vi "ACT_Loop.vi"() -> ()   [LabVIEW 2023, in "Feeder_ACT.lvlib"]
uses:
  Feeder_ACT.lvlib
  Cluster_CMD_ACT_Data.ctl
  ENUM_CMD Mode.ctl
  ENUM_ACT_State.ctl
  <vilib>/Rock Robotics/WPI/PWM/Servo/WPI_ServoDeviceRef.ctl
  <vilib>/Rock Robotics/SystemInterfaces/DIO/FPGA_DIOPWMChannel.ctl
  <vilib>/Rock Robotics/WPI/PWM/WPI_PWMDeadband.ctl
  <vilib>/Rock Robotics/WPI/MotorControl/WPI_MotorControlDeviceRef.ctl
  <vilib>/Rock Robotics/WPI/MotorControl/WPI_MotorControlType.ctl
  <vilib>/Rock Robotics/SystemInterfaces/DIO/FPGA_DIOChannel.ctl
  <vilib>/Rock Robotics/WPI/DigitalInput/WPI_DigitalInputDevRef.ctl
  Shared Code/TypeDefs/ENUM RB_Feeder State.ctl
  ENUM_ACT_Action.ctl
  <vilib>/Rock Robotics/WPI/MotorControl/WPI_MotorControlOpen VictorSP.vi
  RoboRIO Utilities/Global_STOP.vi
  Global_CMD_ACT_Data In.vi
  Tube Wheel/Global_ACT_Data Out.vi
  Global_ACT_Data Out.vi
  Tube Wheel/Tube Wheel_ACT.lvlib
panel:
  out "State":T1
  out "Tube Wheel Ready":bool
  out "Puller Speed (0-1)":dbl
  out "Back":bool
  out "Input DBL Data":T2
  out "Pusher Position (0-100)":dbl
  out "Cycle Time (S)":dbl format="%.3g"
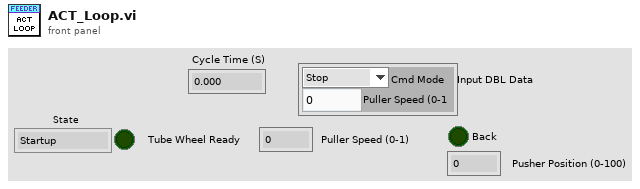
[diagram p1: front panel]
types:
  T1 = typedef "Feeder_ACT.lvlib/ENUM_ACT_State.ctl" = enum16{"Startup", "Back Waiting", "Push Feeding", "Retracting", "Shutdown"}
  T2 = typedef "Feeder_ACT.lvlib/Cluster_CMD_ACT_Data.ctl" = cluster{"Cmd Mode":T3, "Puller Speed (0-1":dbl}
  T3 = typedef "Feeder_ACT.lvlib/ENUM_CMD Mode.ctl" = enum16{"Stop", "Feed Pos 1", "Feed Pos 2", "Fead Full", "Back"}
  T4 = typedef "ENUM RB_Feeder State.ctl" = enum32{"Back", "Reversing", "Shooting"}
  T5 = typedef "WPI_DigitalInputDevRef.ctl" = cluster{"DevStatus":errorcluster, "DIO Channel":T6}
  T6 = typedef "FPGA_DIOChannel.ctl" = enum8{"DIO 0", "DIO 1", "DIO 2", "DIO 3", "DIO 4", "DIO 5", "DIO 6", "DIO 7", "DIO 8", "DIO 9", "DIO MXP 0", "DIO MXP 1", "DIO MXP 2", "DIO MXP 3", "DIO MXP 4", "DIO MXP 5", "DIO MXP 6", "DIO MXP 7", "DIO MXP 8", "DIO MXP 9", "DIO MXP 10", "DIO MXP 11", "DIO MXP 12", "DIO MXP 13", "DIO MXP 14", "DIO MXP 15", "SPI Port CS1", "SPI Port CS2", "SPI Port CS3", "SPI Port MISO", "SPI Port MOSI", "Invalid"}
  T7 = typedef "WPI_MotorControlDeviceRef.ctl" = cluster{"DeviceStatus":errorcluster, "Type":T8, "PWM":cluster{"PWM Channel":T9, "DeadBand":T10}, "CAN":cluster{"Device Number":u8, "SetOutput VI Ref":variant, "GetOutput VI Ref":variant, "Enable VI Ref":variant, "Disable VI Ref":variant, "Data":variant}, "Invert":bool, "DIO PWM":cluster{"PWM \"Enable\" Channel":T9, "DIOChannel":T6, "PWM Rate":dbl}}
  T8 = typedef "WPI_MotorControlType.ctl" = enum16{"PWM", "CAN", "DIO PWM"}
  T9 = typedef "FPGA_DIOPWMChannel.ctl" = enum8{"PWM 0", "PWM 1", "PWM 2", "PWM 3", "PWM 4", "PWM 5", "PWM 6", "PWM 7", "PWM 8", "PWM 9", "PWM MXP 0", "PWM MXP 1", "PWM MXP 2", "PWM MXP 3", "PWM MXP 4", "PWM MXP 5", "PWM MXP 6", "PWM MXP 7", "PWM MXP 8", "PWM MXP 9", "Invalid"}
  T10 = typedef "WPI_PWMDeadband.ctl" = cluster{"Name":string, "maxPositivePwm":i32, "minPositivePwm":i32, "centerPwm":i32, "maxNegativePwm":i32, "minNegativePwm":i32, "angularRange":u16}
  T11 = typedef "WPI_ServoDeviceRef.ctl" = cluster{"DeviceStatus":errorcluster, "PWM Channel":T9, "DeadBand":T10}
  T12 = typedef "Feeder_ACT.lvlib/ENUM_ACT_Action.ctl" = enum16{"No Action", "Reset Time", "Reset All", "Retract Back", "Set Push 1", "Set Push 2", "Set Push 3"}
  T13 = cluster{"PusherServo Ref":T11, "LeftMotor Puller Ref":T7, "RightMotor Puller Ref":T7, "PusherBack Ref":T5, "State":T1, "Previous State":T1, "Current Time":timestamp, "Previous Time":timestamp, "Start Time":timestamp, "Target Time (ms)":u32, "Cycle Time(S)":dbl, "ACT Input":T2, "Pusher Positon(0-100)":dbl, "Puller Speed (0-1)":dbl, "PusherIsBack":bool, "Feeder Display":T4, "Tube Wheel Ready":bool}
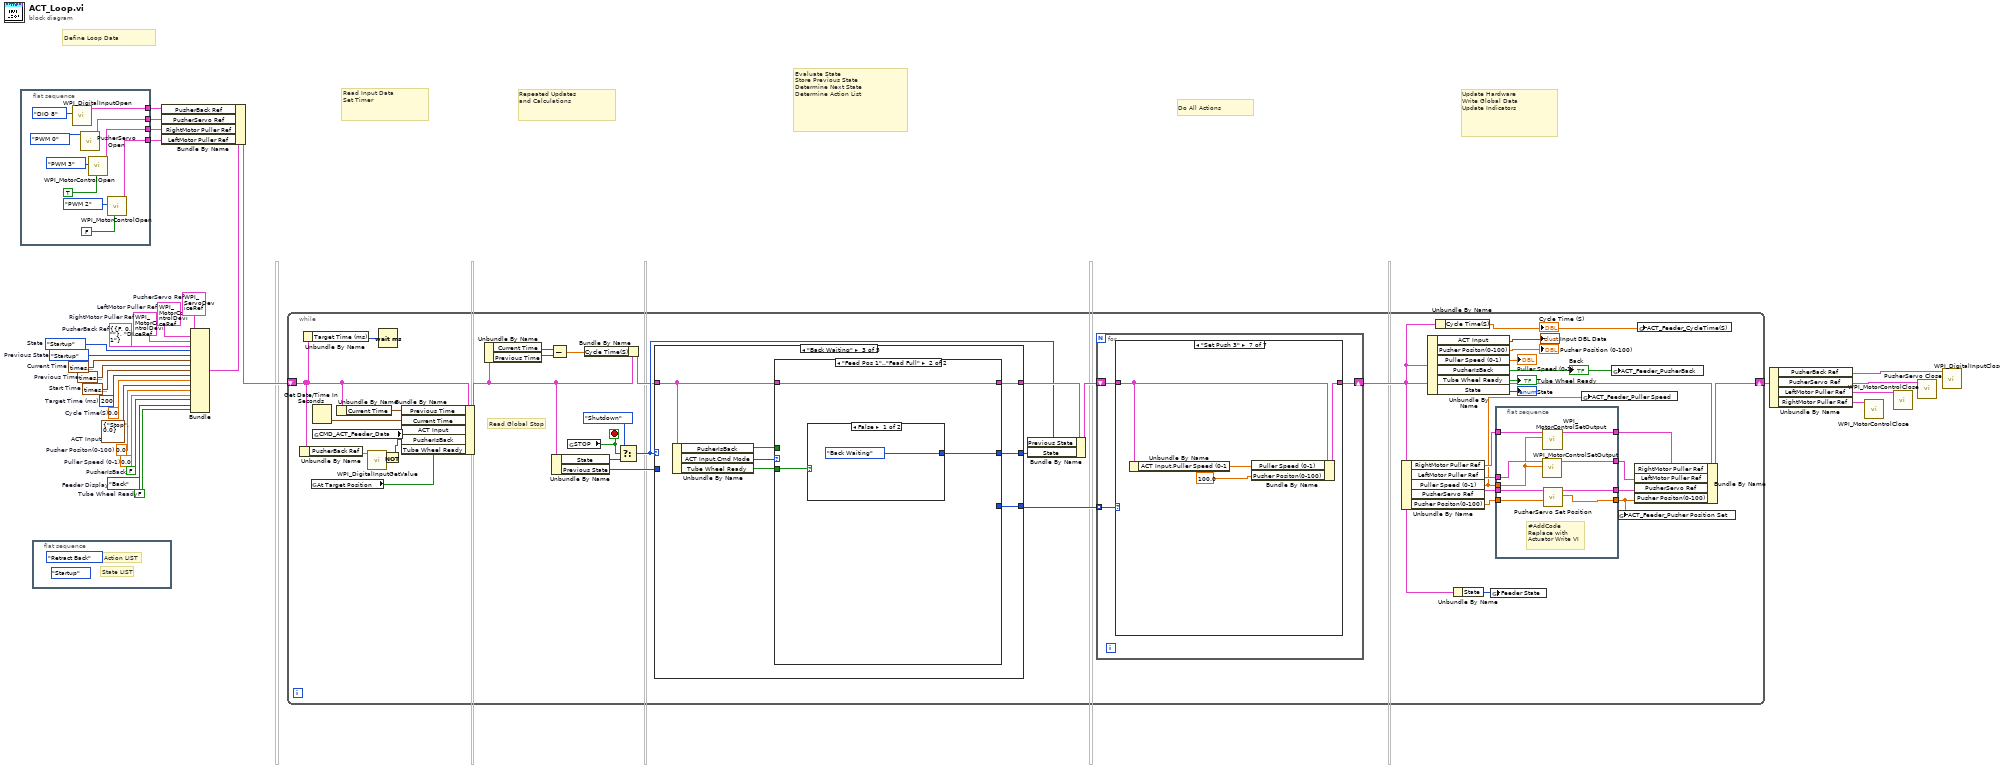
[diagram p0: block diagram]
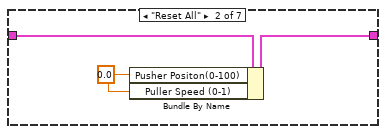
[diagram p3: hidden frame]
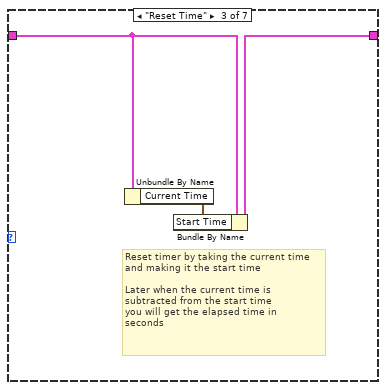
[diagram p4: hidden frame]
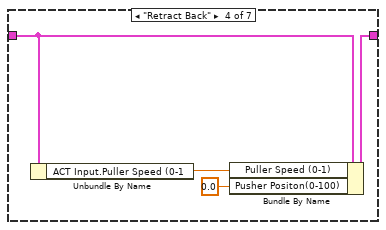
[diagram p5: hidden frame]
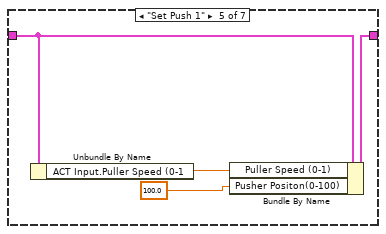
[diagram p6: hidden frame]
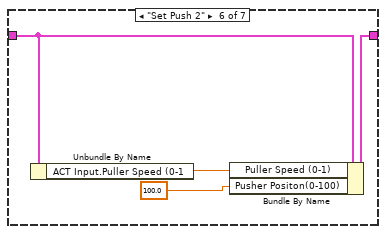
[diagram p7: hidden frame]
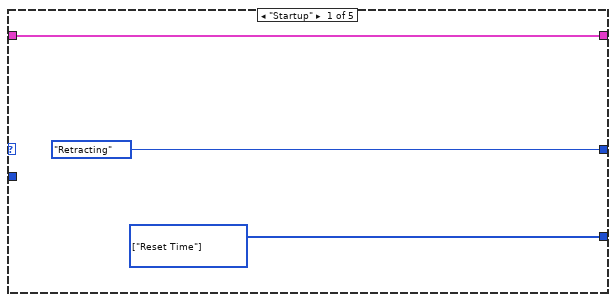
[diagram p8: hidden frame]
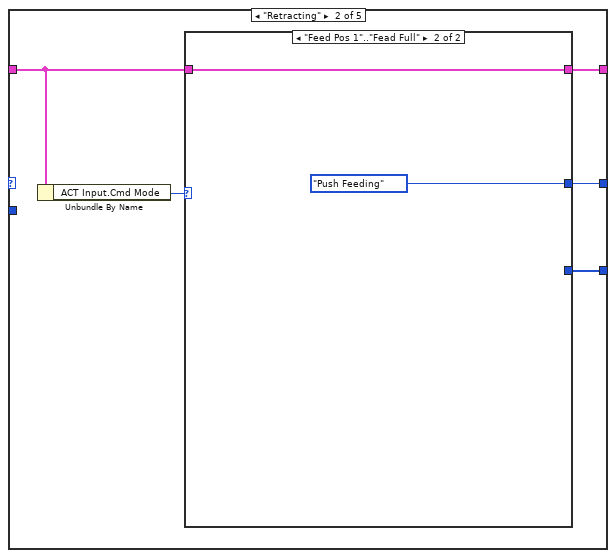
[diagram p9: hidden frame]
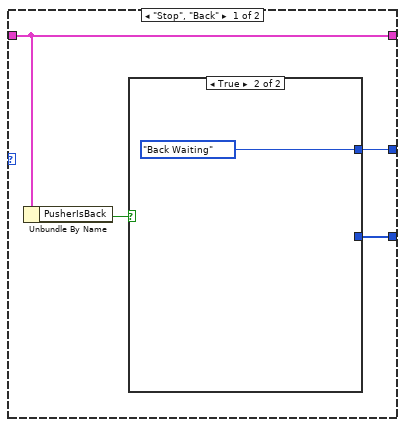
[diagram p10: hidden frame]
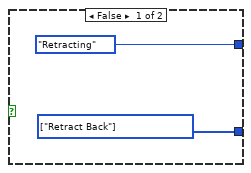
[diagram p11: hidden frame]
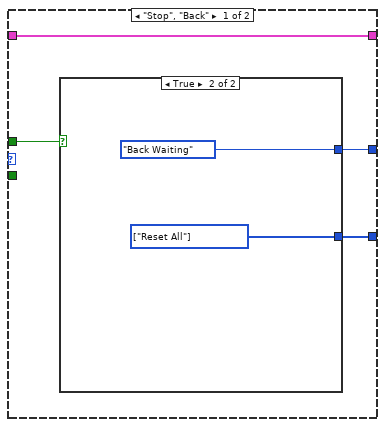
[diagram p12: hidden frame]
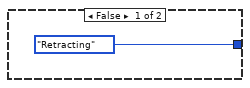
[diagram p13: hidden frame]
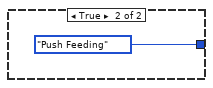
[diagram p14: hidden frame]
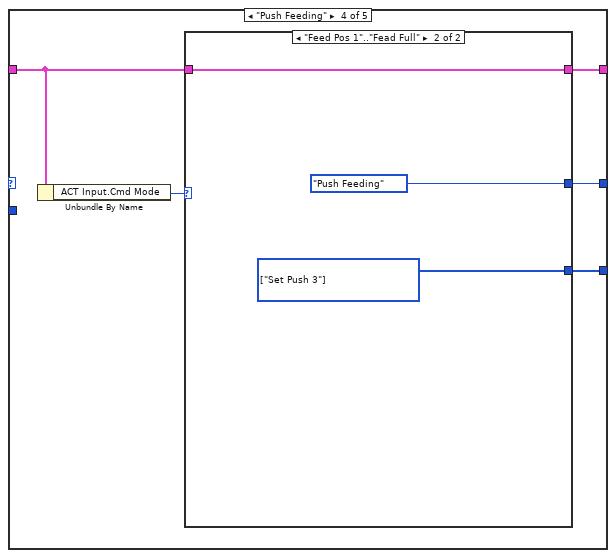
[diagram p15: hidden frame]
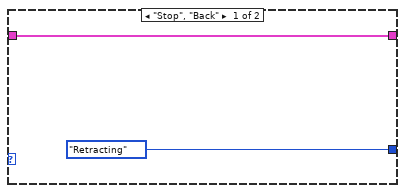
[diagram p16: hidden frame]
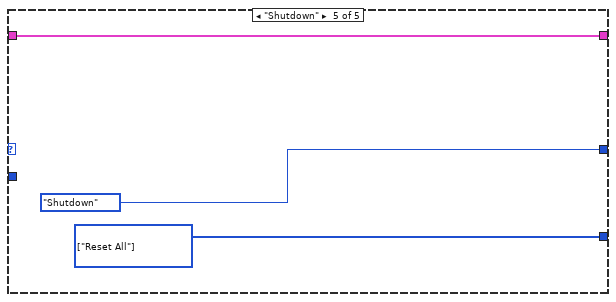
[diagram p17: hidden frame]
diagram:
  w1 = FALSE  # Tube Wheel Ready
  w2 = ENUM_RB_Feeder_State."Back"  # Feeder Display
  w4 = FALSE  # PusherIsBack
  w6 = T5 {"DevStatus"={"status"=FALSE, "code"=0, "source"=""}, "DIO Channel"=enum."DIO 1"}  # PusherBack Ref
  w7 = 0.0  # Puller Speed (0-1)
  w13 = T7 {"DeviceStatus"={"status"=FALSE, "code"=0, "source"=""}, "Type"=enum."PWM", "PWM"={"PWM Channel"=enum."Invalid", "DeadBand"={"Name"="", "maxPositivePwm"=0, "minPositivePwm"=0, "centerPwm"=0, "maxNegativePwm"=0, "minNegativePwm"=0, "angularRange"=0}}, "CAN"={"Device Number"=0, "SetOutput VI Ref"=variant(refnum<vi> refnum), "GetOutput VI Ref"=variant(refnum<vi> refnum), "Enable VI Ref"=variant(refnum<vi> refnum), "Disable VI Ref"=variant(refnum<vi> refnum), "Data"=variant}, "Invert"=FALSE, "DIO PWM"={"PWM \"Enable\" Channel"=enum."Invalid", "DIOChannel"=enum."Invalid", "PWM Rate"=0.0}}  # RightMotor Puller Ref
  w12 = T7 {"DeviceStatus"={"status"=FALSE, "code"=0, "source"=""}, "Type"=enum."PWM", "PWM"={"PWM Channel"=enum."Invalid", "DeadBand"={"Name"="", "maxPositivePwm"=0, "minPositivePwm"=0, "centerPwm"=0, "maxNegativePwm"=0, "minNegativePwm"=0, "angularRange"=0}}, "CAN"={"Device Number"=0, "SetOutput VI Ref"=variant(refnum<vi> refnum), "GetOutput VI Ref"=variant(refnum<vi> refnum), "Enable VI Ref"=variant(refnum<vi> refnum), "Disable VI Ref"=variant(refnum<vi> refnum), "Data"=variant}, "Invert"=FALSE, "DIO PWM"={"PWM \"Enable\" Channel"=enum."Invalid", "DIOChannel"=enum."Invalid", "PWM Rate"=0.0}}  # LeftMotor Puller Ref
  w15 = T11 {"DeviceStatus"={"status"=FALSE, "code"=0, "source"=""}, "PWM Channel"=enum."Invalid", "DeadBand"={"Name"="", "maxPositivePwm"=0, "minPositivePwm"=0, "centerPwm"=0, "maxNegativePwm"=0, "minNegativePwm"=0, "angularRange"=0}}  # PusherServo Ref
  w20 = 0.0  # Cycle Time(S)
  w21 = ENUM_ACT_State."Startup"  # Previous State
  w22 = timestamp(0 s since 1904-01-01)  # Previous Time
  w23 = u32 200  # Target Time (ms)
  w24 = 0.0  # Pusher Positon(0-100)
  w25 = T2 {"Cmd Mode"=enum."Stop", "Puller Speed (0-1"=0.0}  # ACT Input
  w26 = timestamp(0 s since 1904-01-01)  # Start Time
  w27 = timestamp(0 s since 1904-01-01)  # Current Time
  w28 = ENUM_ACT_State."Startup"  # State
  # "Define Loop Data"
  # "Repeated Updates\nand Calculations"
  # "Read Input Data\nSet Timer"
  # "Evaluate State\nStore Previous State\nDetermine Next State\nDetermine Action List"
  # "Do All Actions"
  # "Update Hardware\nWrite Global Data\nUpdate Indicators"
  n1 = flat-sequence {
    tunnel: [w37] -> w16
    tunnel: [w34] -> w11
    tunnel: [w31] -> w10
    tunnel: [w30] -> w5
    frame #0 {
      n2 = call <vilib>:"WPI_DigitalInputOpen.vi"("DIO Channel"=FPGA_DIOChannel."DIO 8") -> ("DigitalInputDevRef"=w30:T5)  [unwired: 9 in, 1 out]
      n3 = call "PusherServo Open.vi"("PWM Channel"=FPGA_DIOPWMChannel."PWM 0") -> ("ServoDeviceRef Out"=w37:T11)  [unwired: 9 in, 1 out]
      n4 = call-poly <vilib>:"WPI_MotorControlOpen.vi"("Invert"=TRUE, "PWM Channel"=FPGA_DIOPWMChannel."PWM 3") -> ("MotorControlDeviceRef"=w34:T7)  [unwired: 8 in, 1 out]
      n5 = call-poly <vilib>:"WPI_MotorControlOpen.vi"("Invert"=FALSE, "PWM Channel"=FPGA_DIOPWMChannel."PWM 2") -> ("MotorControlDeviceRef"=w31:T7)  [unwired: 8 in, 1 out]
    }
  }
  n6 = flat-sequence {
    frame #0 {
      (unwired) ENUM_ACT_State."Startup" ("State")
      (unwired) ENUM_ACT_Action."Retract Back" ("Action")
      # "State LIST"
      # "Action LIST"
    }
  }
  n7 = Bundle("PusherServo Ref"=w15, "LeftMotor Puller Ref"=w12, "RightMotor Puller Ref"=w13, "PusherBack Ref"=w6, "State"=w28, "Previous State"=w21, "Current Time"=w27, "Previous Time"=w22, "Start Time"=w26, "Target Time (ms)"=w23, "Cycle Time(S)"=w20, "ACT Input"=w25, "Pusher Positon(0-100)"=w24, "Puller Speed (0-1)"=w7, "PusherIsBack"=w4, "Feeder Display"=w2, "Tube Wheel Ready"=w1) -> (w18:T13)  [unwired: 1 in]
  n8 = Bundle By Name(cluster=w18, "PusherBack Ref"=w5, "PusherServo Ref"=w16, "RightMotor Puller Ref"=w11, "LeftMotor Puller Ref"=w10) -> (w17:T13)
  n9 = while {
    shift-right: [w58] -> w19
    shift-left: w17 -> [w50]
    stop <- w76 stop-if-true
    # "Read Global Stop"
    n10 = Unbundle By Name(w50) -> ("PusherBack Ref"=w49:T5)
    n11 = Unbundle By Name(w50) -> ("Target Time (ms)"=w73:u32)
    n12 = global read "Global_ACT_Data Out.vi" "At Target Position"() -> (w41:bool)
    n13 = Get Date/Time In Seconds() -> (seconds since 1Jan1904=w80:timestamp)
    n14 = global read "Global_CMD_ACT_Data In.vi" "CMD_ACT_Feeder_Data"() -> (w61:T2)
    n15 = Unbundle By Name(w50) -> ("Current Time"=w72:timestamp)
    n16 = call <vilib>:"WPI_DigitalInputGetValue.vi"("DigitalInputDevRef"=w49) -> ("Value"=w48:bool)  [unwired: 8 in, 2 out]
    n17 = Wait (ms)(milliseconds to wait=w73) -> ()  [unwired: 1 out]
    n18 = Not(x=w48) -> (.not. x?=w47:bool)
    n19 = Bundle By Name(cluster=w50, "Previous Time"=w72, "Current Time"=w80, "ACT Input"=w61, "PusherIsBack"=w47, "Tube Wheel Ready"=w41) -> (w66:T13)
    n20 = Unbundle By Name(w66) -> ("Current Time"=w67:timestamp, "Previous Time"=w68:timestamp)
    n21 = Subtract(x=w67, y=w68) -> (x-y=w64:dbl)
    n22 = Unbundle By Name(w66) -> ("State"=w74:T1, "Previous State"=w71:T1)
    n23 = global read "Global_STOP.vi" "STOP"() -> (w76:bool)
    n24 = Bundle By Name(cluster=w66, "Cycle Time(S)"=w64) -> (w65:T13)
    n25 = Select(t=ENUM_ACT_State."Shutdown" ("State"), s=w76, f=w74) -> (s? t:f=w69:T1)
    n26 = case shown="\"Back Waiting\"" w69 {
      tunnel: w65 -> [w118 w121 w137 w154 w164]
      tunnel: [w118 w120 w136 w153 w164] -> w78
      tunnel: [ENUM_ACT_State."Retracting" ("State") w123 w139 w156 ENUM_ACT_State."Shutdown" ("State")] -> w77
      tunnel: [w117 w119 w135 w152 w162] -> w63
      tunnel: w71 -> [_ _ _ _ _]
      frame "Startup" {
        w117 = T12[] [enum."Reset Time"] items=["No Action", "Reset Time", "Reset All", "Retract Back", "Set Push 1", "Set Push 2", "Set Push 3"] ("Actions")
      }
      frame "Retracting" {
        n27 = Unbundle By Name(w121) -> ("ACT Input.Cmd Mode"=w122:T3)
        n28 = case shown="\"Feed Pos 1\"..\"Fead Full\"" w122 {
          tunnel: [w127 ENUM_ACT_State."Push Feeding" ("State")] -> w123
          tunnel: w121 -> [w126 w131]
          tunnel: [w126 w131] -> w120
          tunnel: [w124 _] -> w119
          frame "Stop", "Back" {
            n29 = Unbundle By Name(w126) -> ("PusherIsBack"=w125:bool)
            n30 = case shown="True" w125 {
              tunnel: [ENUM_ACT_State."Retracting" ("State") ENUM_ACT_State."Back Waiting" ("State")] -> w127
              tunnel: [w128 _] -> w124
              frame False {
                w128 = T12[] [enum."Retract Back"] items=["No Action", "Reset Time", "Reset All", "Retract Back", "Set Push 1", "Set Push 2", "Set Push 3"] ("Actions")
              }
              frame True {
              }
            }
          }
          frame "Feed Pos 1".."Fead Full" {
          }
        }
      }
      frame "Back Waiting" {
        n31 = Unbundle By Name(w137) -> ("PusherIsBack"=w134:bool, "ACT Input.Cmd Mode"=w138:T3, "Tube Wheel Ready"=w133:bool)
        n32 = case shown="\"Feed Pos 1\"..\"Fead Full\"" w138 {
          tunnel: [w143 w149] -> w139
          tunnel: w137 -> [w142 w148]
          tunnel: [w142 w148] -> w136
          tunnel: [w141 _] -> w135
          tunnel: w134 -> [w140 _]
          tunnel: w133 -> [_ w147]
          frame "Stop", "Back" {
            n33 = case shown="True" w140 {
              tunnel: [ENUM_ACT_State."Retracting" ("State") ENUM_ACT_State."Back Waiting" ("State")] -> w143
              tunnel: [_ w145] -> w141
              frame False {
              }
              frame True {
                w145 = T12[] [enum."Reset All"] items=["No Action", "Reset Time", "Reset All", "Retract Back", "Set Push 1", "Set Push 2", "Set Push 3"] ("Actions")
              }
            }
          }
          frame "Feed Pos 1".."Fead Full" {
            n34 = case shown="False" w147 {
              tunnel: [ENUM_ACT_State."Back Waiting" ("State") ENUM_ACT_State."Push Feeding" ("State")] -> w149
              frame False {
              }
              frame True {
              }
            }
          }
        }
      }
      frame "Push Feeding" {
        n35 = Unbundle By Name(w154) -> ("ACT Input.Cmd Mode"=w155:T3)
        n36 = case shown="\"Feed Pos 1\"..\"Fead Full\"" w155 {
          tunnel: [ENUM_ACT_State."Retracting" ("State") ENUM_ACT_State."Push Feeding" ("State")] -> w156
          tunnel: w154 -> [w158 w160]
          tunnel: [w158 w160] -> w153
          tunnel: [_ w159] -> w152
          frame "Stop", "Back" {
          }
          frame "Feed Pos 1".."Fead Full" {
            w159 = T12[] [enum."Set Push 3"] items=["No Action", "Reset Time", "Reset All", "Retract Back", "Set Push 1", "Set Push 2", "Set Push 3"] ("Actions")
          }
        }
      }
      frame "Shutdown" {
        w162 = T12[] [enum."Reset All"] items=["No Action", "Reset Time", "Reset All", "Retract Back", "Set Push 1", "Set Push 2", "Set Push 3"] ("Actions")
      }
    }
    n37 = Bundle By Name(cluster=w78, "Previous State"=w69, "State"=w77) -> (w79:T13)
    n38 = for {
      tunnel: w63 -> [w92] mode=indexing
      shift-right: [w91] -> w43
      shift-left: w79 -> [w90]
      n39 = case shown="\"Set Push 3\"" w92 {
        tunnel: w90 -> [w93 w96 w99 w102 w106 w110 w114]
        tunnel: [w93 w95 w98 w103 w107 w111 w115] -> w91
        frame "No Action" {
        }
        frame "Reset All" {
          w94 = 0.0 ("FG Write Value")
          n40 = Bundle By Name(cluster=w96, "Pusher Positon(0-100)"=w94, "Puller Speed (0-1)"=w94) -> (w95:T13)
        }
        frame "Reset Time" {
          # "Reset timer by taking the current time\nand making it the start time\n\nLater when the current time is \nsubtracted from the start time\nyou will get the elapsed time in \nseconds"
          n41 = Unbundle By Name(w99) -> ("Current Time"=w97:timestamp)
          n42 = Bundle By Name(cluster=w99, "Start Time"=w97) -> (w98:T13)
        }
        frame "Retract Back" {
          n43 = Unbundle By Name(w102) -> ("ACT Input.Puller Speed (0-1"=w101:dbl)
          n44 = Bundle By Name(cluster=w102, "Puller Speed (0-1)"=w101, "Pusher Positon(0-100)"=0.0) -> (w103:T13)
        }
        frame "Set Push 1" {
          n45 = Unbundle By Name(w106) -> ("ACT Input.Puller Speed (0-1"=w105:dbl)
          n46 = Bundle By Name(cluster=w106, "Puller Speed (0-1)"=w105, "Pusher Positon(0-100)"=100.0) -> (w107:T13)
        }
        frame "Set Push 2" {
          n47 = Unbundle By Name(w110) -> ("ACT Input.Puller Speed (0-1"=w109:dbl)
          n48 = Bundle By Name(cluster=w110, "Puller Speed (0-1)"=w109, "Pusher Positon(0-100)"=100.0) -> (w111:T13)
        }
        frame "Set Push 3" {
          n49 = Unbundle By Name(w114) -> ("ACT Input.Puller Speed (0-1"=w113:dbl)
          n50 = Bundle By Name(cluster=w114, "Puller Speed (0-1)"=w113, "Pusher Positon(0-100)"=100.0) -> (w115:T13)
        }
      }
    }
    n51 = Unbundle By Name(w43) -> ("RightMotor Puller Ref"=w54:T7, "LeftMotor Puller Ref"=w53:T7, "Puller Speed (0-1)"=w46:dbl, "PusherServo Ref"=w60:T11, "Pusher Positon(0-100)"=w56:dbl)
    n52 = Unbundle By Name(w43) -> ("ACT Input"=→"Input DBL Data":T2, "Pusher Positon(0-100)"=→"Pusher Position (0-100)":dbl, "Puller Speed (0-1)"=→"Puller Speed (0-1)":dbl, "PusherIsBack"=w44:bool, "Tube Wheel Ready"=→"Tube Wheel Ready":bool, "State"=→"State":T1)
    "Back" <- w44
    n53 = Unbundle By Name(w43) -> ("Cycle Time(S)"=w57:dbl)
    "Cycle Time (S)" <- w57
    n54 = Unbundle By Name(w43) -> ("State"=w42:T1)
    n55 = global write "Global_ACT_Data Out.vi" "Feeder State"(w42) -> ()
    n56 = flat-sequence {
      tunnel: w60 -> [w88]
      tunnel: [w89] -> w59
      tunnel: w56 -> [w87]
      tunnel: [w81] -> w55
      tunnel: w54 -> [w86]
      tunnel: w53 -> [w85]
      tunnel: [w84] -> w52
      tunnel: [w83] -> w51
      tunnel: w46 -> [w82]
      frame #0 {
        # "#AddCode\nReplace with\nActuator Write VI"
        n57 = call <vilib>:"WPI_MotorControlSetOutput.vi"("Output"=w82, "MotorControlDevRef"=w85) -> ("MotorControlDevRef"=w83:T7)  [unwired: 7 in, 2 out]
        n58 = call <vilib>:"WPI_MotorControlSetOutput.vi"("Output"=w82, "MotorControlDevRef"=w86) -> ("MotorControlDevRef"=w84:T7)  [unwired: 7 in, 2 out]
        n59 = call "PusherServo Set Position.vi"("Stroke (0-100)"=w87, "ServoDeviceRef"=w88) -> ("Stroke Set"=w81:dbl, "ServoDeviceRef Out"=w89:T11)  [unwired: 7 in, 1 out]
      }
    }
    n60 = global write "Global_ACT_Data Out.vi" "ACT_Feeder_Puller Speed"(w46) -> ()
    n61 = global write "Global_ACT_Data Out.vi" "ACT_Feeder_PusherBack"(w44) -> ()
    n62 = global write "Global_ACT_Data Out.vi" "ACT_Feeder_Pusher Position Set"(w55) -> ()
    n63 = Bundle By Name(cluster=w43, "RightMotor Puller Ref"=w52, "LeftMotor Puller Ref"=w51, "PusherServo Ref"=w59, "Pusher Positon(0-100)"=w55) -> (w58:T13)
    n64 = global write "Global_ACT_Data Out.vi" "ACT_Feeder_CycleTime(S)"(w57) -> ()
  }
  n65 = Unbundle By Name(w19) -> ("PusherBack Ref"=w3:T5, "PusherServo Ref"=w14:T11, "LeftMotor Puller Ref"=w9:T7, "RightMotor Puller Ref"=w8:T7)
  n66 = call <vilib>:"WPI_MotorControlClose.vi"("MotorControlDevRef"=w8) -> ()  [unwired: 10 in, 1 out]
  n67 = call <vilib>:"WPI_MotorControlClose.vi"("MotorControlDevRef"=w9) -> ()  [unwired: 10 in, 1 out]
  n68 = call "PusherServo Close.vi"("ServoDeviceRef Out"=w14) -> ()  [unwired: 10 in, 1 out]
  n69 = call <vilib>:"WPI_DigitalInputClose.vi"("DigitalInputDevRef"=w3) -> ()  [unwired: 10 in, 1 out]
